vi "TrajectoryConfig_GetMaxVelAccel.vi"(11 "inTRAJECTORY_CONFIG":T1 {"End Velocity" format="%20.4f"; "StartVelocity" format="%20.4f"; "Max Acceleration" format="%20.4f"; "MaxVelocity" format="%20.4f"}) -> (1 "Max Acceleration":dbl, 3 "MaxVelocity":dbl)   [LabVIEW 2019, in "Trajectory_Library.lvlib"]
doc: "Retrieves the Maximum Velocity and Acceleration from the Trajectory Configuration.\n\nParameters:\n - InTrajectoryConfig -- The trajectory configuration data structure\n\nReturns:\n - Maximum Velocity -- Maximum velocity defined in configuration\n - Maximum Acceleration -- Maximum acceleration defined in configuration."
uses:
  Trajectory_Library.lvlib
  TypeDef/TRAJ_CONFIG.ctl
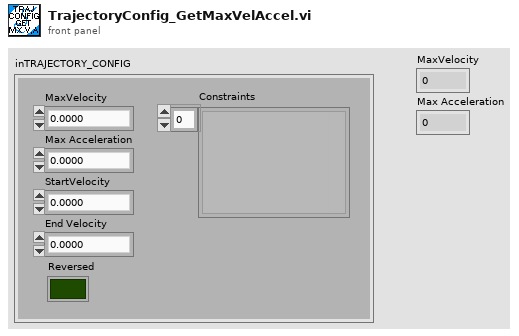
[diagram p1: front panel]
types:
  T1 = typedef "Trajectory_Library.lvlib/TRAJ_CONFIG.ctl" = cluster{"MaxVelocity":dbl, "Max Acceleration":dbl, "StartVelocity":dbl, "End Velocity":dbl, "Reversed":bool, "Constraints":variant[]}
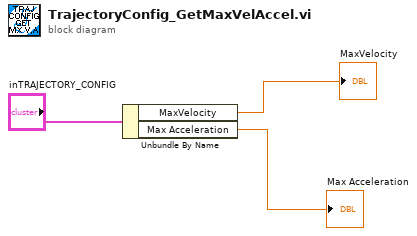
[diagram p0: block diagram]
diagram:
  n1 = Unbundle By Name("inTRAJECTORY_CONFIG") -> ("MaxVelocity"=→"MaxVelocity":dbl, "Max Acceleration"=→"Max Acceleration":dbl)
